vi "grab.vi"() -> ()   [LabVIEW 2011]
uses:
  <userlib>/labvvis/New Image/New Image (RGBA).vi
  <userlib>/labvvis/labvvis.lvlib
panel:
  out "Error":string
  in  "stop":bool
  out "Output":picture
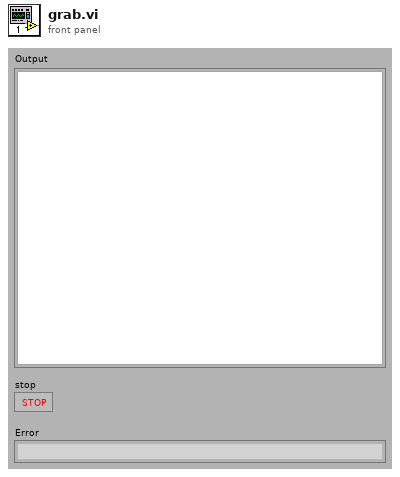
[diagram p1: front panel]
types:
  T1 = typedef "labvvis.lvlib/VVIS Image.ctl" = cluster{"Image ID":i16, "Channel ID":i16}
  T2 = typedef "imagedata.ctl" = cluster{"image type":i32, "image depth":i32, "image":u8[], "mask":u8[], "colors":u32[], "Rectangle":cluster{"left":i16, "top":i16, "right":i16, "bottom":i16}}
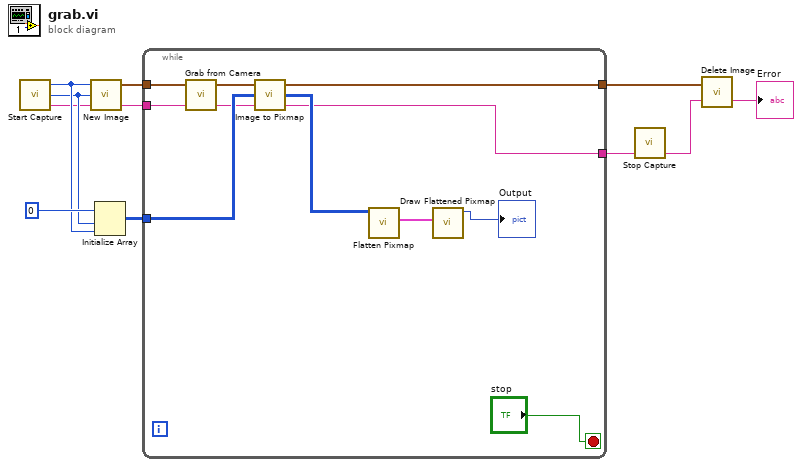
[diagram p0: block diagram]
diagram:
  n1 = call <userlib>:"Start Capture.vi"() -> ("Error"=w4:string, "Height"=w5:i32, "Width"=w6:i32)  [unwired: 3 in]
  n2 = call-poly <userlib>:"New Image.vi"("Error"=w4, "Height"=w5, "Width"=w6) -> ("Error"=w7:string, "VVIS Image"=w8:T1)  [unwired: 1 in]
  n3 = Initialize Array(0, w5, w6) -> (w10:i32[][])
  n4 = while {
    tunnel: w10 -> [w21]
    tunnel: [w19] -> w9
    tunnel: w8 -> [w18]
    tunnel: w7 -> [w15]
    tunnel: [w14] -> w3
    stop <- "stop" stop-if-true
    n5 = call <userlib>:"Grab from Camera.vi"("Error"=w15, "Image"=w18) -> ("Error"=w16:string, "Image"=w17:T1)  [unwired: 1 in, 1 out]
    n6 = call <userlib>:"Image to Pixmap.vi"("Error"=w16, "Output Pixmap"=w21, "Image"=w17) -> ("Error"=w14:string, "Output Pixmap"=w20:u32[][], "Image"=w19:T1)
    n7 = call <vilib>:"Flatten Pixmap.vi"("24-bit pixmap"=w20) -> ("image data"=w22:T2)  [unwired: 10 in]
    n8 = call <vilib>:"Draw Flattened Pixmap.vi"("image data"=w22) -> ("new picture"=→"Output":picture)  [unwired: 8 in]
  }
  n9 = call <userlib>:"Stop Capture.vi"("Error"=w3) -> ("Error"=w2:string)  [unwired: 4 in]
  n10 = call <userlib>:"Delete Image.vi"("Error"=w2, "Image"=w9) -> ("Error"=→"Error":string)  [unwired: 1 in]
